vi "Test Multipart Request.vi"() -> ()   [LabVIEW 2020]
uses:
  HTTP Utils/Request/Request.lvclass
  HTTP Utils/FormField/FormField.lvclass
  lv-uri/URI/URI/URI.lvclass
  HTTP Utils/Method.ctl
  HTTP Utils/HTTP Utils.lvlib
panel:
  out "Form Fields":T1(array[cluster])
  out "Is Form?":bool
  out "Error":errorcluster
  out "Method":T2
  out "Target":string="/hello.htm"
  out "Version String":string="HTTP/1.1"
  out "Headers":cluster{"Header":string, "Value":string}[](array[cluster])=[{"Header"="accept-encoding", "Value"="gzip, deflate"}, {"Header"="accept-language", "Value"="en-us"}, {"Header"="connection", "Value"="Keep-Alive"}, {"Header"="host", "Value"="www.tutorialspoint.com"}, {"Header"="user-agent", "Value"="Mozilla/4.0 (compatible; MSIE5.01; Windows NT)"}]
  in  "Listen Port":u16=36987
  # "Name"
  # "File"
  # "MIME Type"
  # "Original Name"
  # "Uploaded Temp Path"
  # "Value (Not Saved File)"
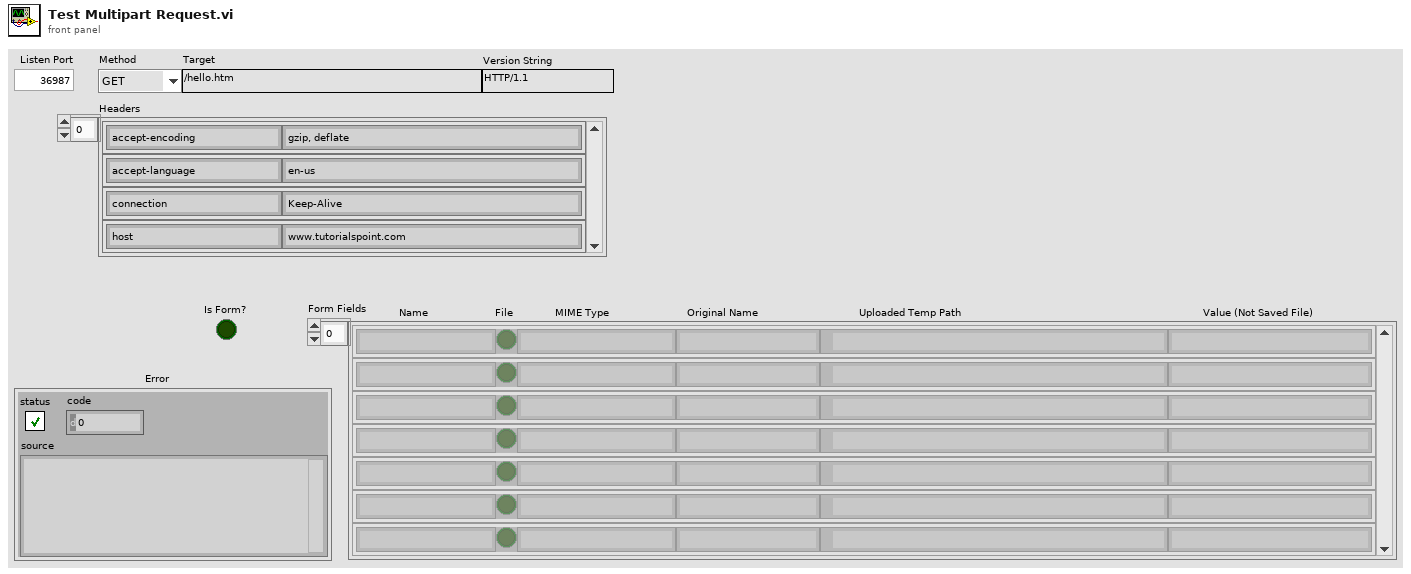
[diagram p1: front panel]
types:
  T1 = cluster{"Name":string, "Is File?":bool, "MIME Type":string, "Original Name":string, "Path":path, "Value":string}[]
  T2 = typedef "HTTP Utils.lvlib/Method.ctl" = enum16{"GET", "HEAD", "POST", "PUT", "DELETE", "CONNECT", "OPTIONS", "TRACE", "PATCH"}
  T3 = cluster{"Properties:Name":string, "Properties:Is File?":bool, "Properties:MIME Type":string, "Properties:Original Name":string, "Properties:Path":path, "Properties:Value":string}
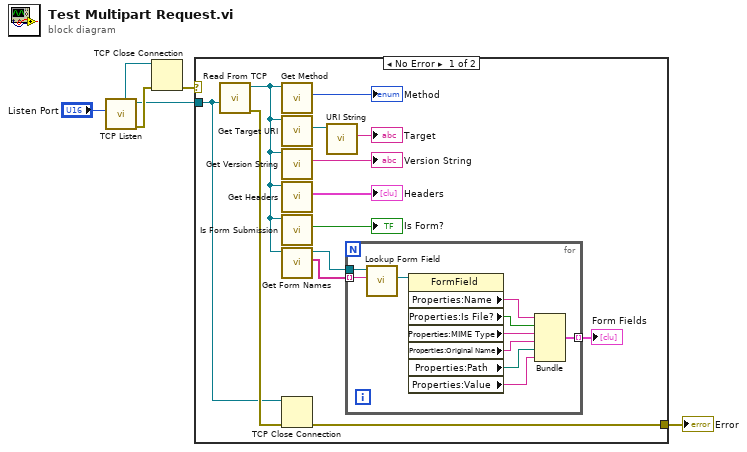
[diagram p0: block diagram]
diagram:
  n1 = call <vilib>:"TCP Listen.vi"("port"="Listen Port") -> ("error out"=w5:errorcluster, "connection ID"=w2:refnum<k5>, "listener ID"=w4:refnum<k5>)  [unwired: 6 in, 2 out]
  n2 = TCP Close Connection(connection ID=w4, error in (no error)=w5) -> (error out=w3:errorcluster)  [unwired: 1 in, 1 out]
  n3 = case shown="No Error" w3 {
    selector: w3 -> [_ w30]
    tunnel: w2 -> [w13 _]
    tunnel: [w12 w30] -> w1
    frame No Error {
      n4 = call "Read From TCP.vi"("TCP Connection"=w13) -> ("error out"=w19:errorcluster, "Request out"=w9:refnum<class "Request.lvclass">)  [unwired: 9 in]
      n5 = call "Get Method.vi"("Request in"=w9) -> ("Method"=→"Method":T2)  [unwired: 8 in, 2 out]
      n6 = call "Get Target URI.vi"("Request in"=w9) -> ("Target URI"=w18:refnum<class "URI.lvclass">)  [unwired: 8 in, 2 out]
      n7 = call "Get Version String.vi"("Request in"=w9) -> ("Version String"=→"Version String":string)  [unwired: 8 in, 2 out]
      n8 = call "Get Headers.vi"("Request in"=w9) -> ("Headers"=→"Headers":cluster{"Header":string, "Value":string}[])  [unwired: 8 in, 2 out]
      n9 = call "Is Form Submission.vi"("Request in"=w9) -> ("Is Form Submission?"=→"Is Form?":bool)  [unwired: 8 in, 2 out]
      n10 = call "Get Form Names.vi"("Request in"=w9) -> ("Form Names"=w10:string[], "Request out"=w7:refnum<class "Request.lvclass">)  [unwired: 8 in, 1 out]
      n11 = TCP Close Connection(connection ID=w13, error in (no error)=w19) -> (error out=w12:errorcluster)  [unwired: 1 in, 1 out]
      n12 = call "URI String.vi"("URI in"=w18) -> ("URI String"=→"Target":string)  [unwired: 9 in, 1 out]
      n13 = for {
        tunnel: w7 -> [w29]
        tunnel: w10 -> [w28] mode=indexing
        tunnel: [w20] -> w8 mode=indexing
        n14 = call "Lookup Form Field.vi"("Name"=w28, "Request in"=w29) -> ("Field"=w27:refnum<class "FormField.lvclass">)  [unwired: 6 in, 3 out]
        n15 = property class="FormField"(reference=w27) -> ("Properties:Name"=w26:string, "Properties:Is File?"=w24:bool, "Properties:MIME Type"=w25:string, "Properties:Original Name"=w23:string, "Properties:Path"=w21:path, "Properties:Value"=w22:string)  [unwired: 1 in, 2 out]
        n16 = Bundle("Properties:Name"=w26, "Properties:Is File?"=w24, "Properties:MIME Type"=w25, "Properties:Original Name"=w23, "Properties:Path"=w21, "Properties:Value"=w22) -> (w20:T3)  [unwired: 1 in]
      }
      "Form Fields" <- w8
    }
    frame Error {
    }
  }
  "Error" <- w1
